vi "Destroy.vi"(8 "error in (no error)":errorcluster, 11 "Ship in":refnum<class "Ship.lvclass">) -> (0 "error out":errorcluster)   [LabVIEW 2021, in "Ship.lvclass"]
uses:
  Ship.lvclass
  Ship.lvclass/Ship.ctl
  Resource Manager/Resource Manager.lvclass
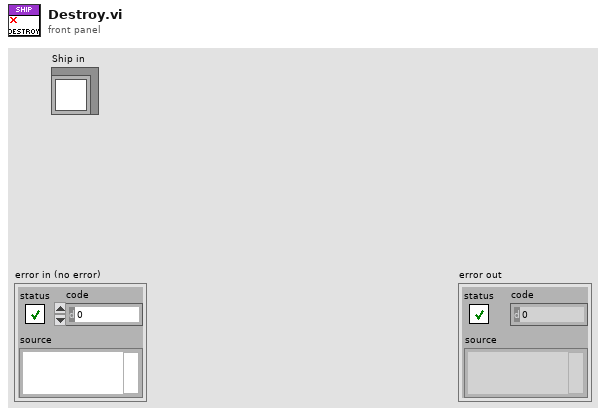
[diagram p1: front panel]
types:
  T1 = cluster{"Primary Weapon":string, "Special Function":string}
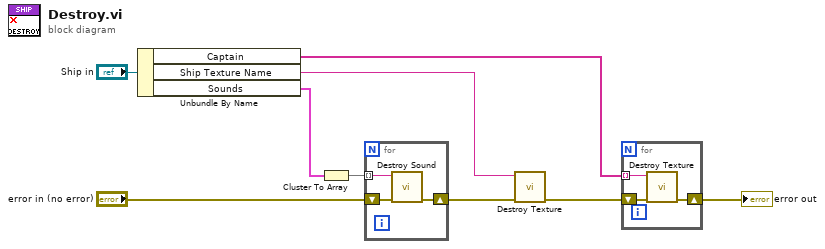
[diagram p0: block diagram]
diagram:
  n1 = Unbundle By Name("Ship in") -> ("Captain"=w6:string[], "Ship Texture Name"=w8:string, "Sounds"=w5:T1)
  n2 = Cluster To Array(cluster=w5) -> (array=w4:string[])
  n3 = for {
    tunnel: w4 -> [w12] mode=indexing
    shift-right: [w10] -> w2
    shift-left: "error in (no error)" -> [w11]
    n4 = call "Destroy Sound.vi"("error in (no error)"=w11, "Texture Name"=w12) -> ("error out"=w10:errorcluster)  [unwired: 9 in]
  }
  n5 = call "Destroy Texture.vi"("error in (no error)"=w2, "Texture Name"=w8) -> ("error out"=w1:errorcluster)  [unwired: 9 in]
  n6 = for {
    shift-right: [w14] -> w7
    shift-left: w1 -> [w15]
    tunnel: w6 -> [w13] mode=indexing
    n7 = call "Destroy Texture.vi"("error in (no error)"=w15, "Texture Name"=w13) -> ("error out"=w14:errorcluster)  [unwired: 9 in]
  }
  "error out" <- w7
